vi "getChannelNames.vi"(8 "error in (no error)":errorcluster, 11 "StaticOutputEditor in":refnum<class "StaticOutputEditor.lvclass">) -> (0 "error out":errorcluster, 2 "channelNames":string[](array[string]), 3 "StaticOutputEditor out":refnum<class "StaticOutputEditor.lvclass">)   [LabVIEW 2009, in "Views.lvlib" / "ScriptEditor.lvlib" / "StaticOutputEditor.lvclass"]
uses:
  StaticOutputEditor.lvclass
  StaticOutputEditor.lvclass/StaticOutputEditor.ctl
  Tools/DatabaseHelpers/Database Objects/ChannelArray/ChannelArray.lvclass
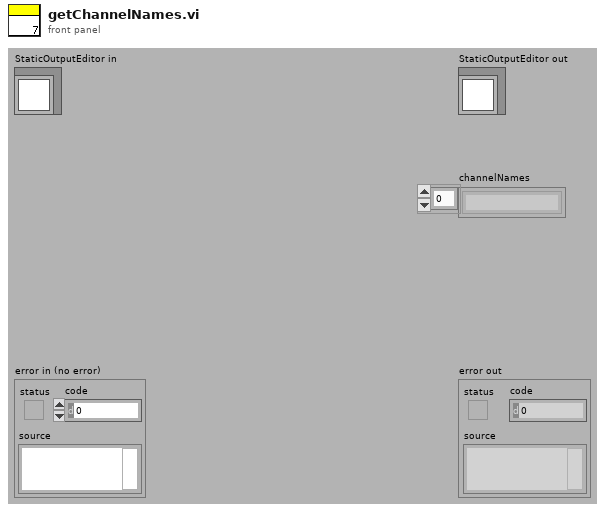
[diagram p1: front panel]
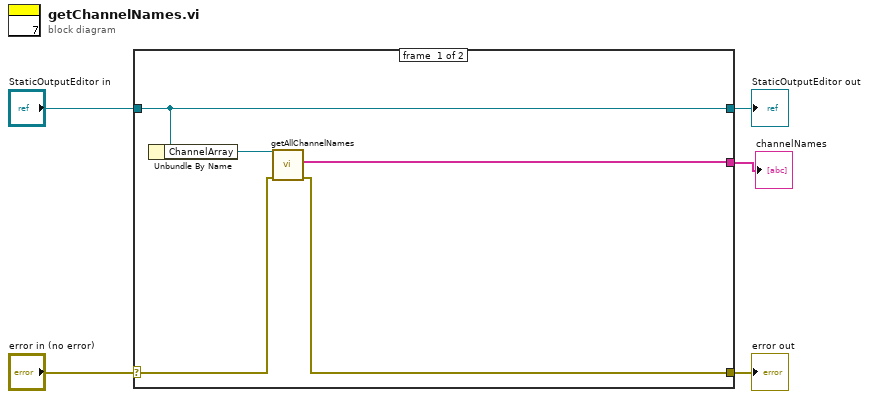
[diagram p0: block diagram]
diagram:
  n1 = case shown="No Error" "error in (no error)" {
    selector: "error in (no error)" -> [w8 w12]
    tunnel: [w7 w12] -> w4
    tunnel: [w10 w11] -> w2
    tunnel: "StaticOutputEditor in" -> [w10 w11]
    tunnel: [w6 _] -> w1
    frame #0 {
      n2 = Unbundle By Name(w10) -> ("ChannelArray"=w9:refnum<class "ChannelArray.lvclass">)
      n3 = call "getAllChannelNames.vi"("error in (no error)"=w8, "ChannelArray in"=w9) -> ("error out"=w7:errorcluster, "channelNames"=w6:string[])  [unwired: 7 in, 1 out]
    }
    frame #1 {
    }
  }
  "error out" <- w4
  "StaticOutputEditor out" <- w2
  "channelNames" <- w1
